vi "Callback - SpeechRecongized.vi"(4 "识别结果":refnum<vi>, 5 "事件数据":T1, 6 "控件引用":refnum<k24>, 7 "事件通用数据":cluster{"源":i32, "类型":u32, "时间":u32}) -> ()   [LabVIEW 2020]
doc: "该回调VI在网页浏览器ActiveX对象上运行Navigate2方法时运行。"
uses:
  System.Speech
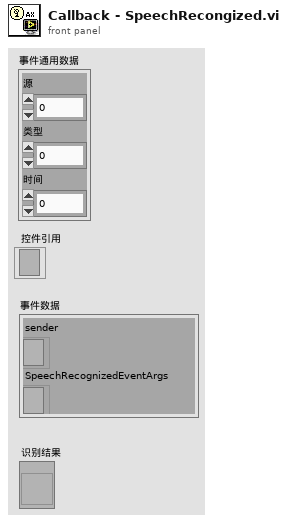
[diagram p1: front panel]
types:
  T1 = cluster{"sender":refnum<k24>, "SpeechRecognizedEventArgs":refnum<k24>}
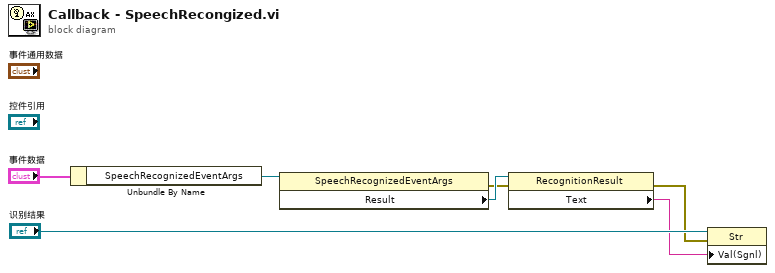
[diagram p0: block diagram]
diagram:
  n1 = Unbundle By Name("事件数据") -> ("SpeechRecognizedEventArgs"=w5:refnum<k24>)
  n2 = property class="SpeechRecognizedEventArgs"(reference=w5) -> (error out=w2:errorcluster, "Result"=w4:refnum<k24>)  [unwired: 1 in, 1 out]
  n3 = property class="RecognitionResult"(reference=w4, error in=w2) -> (error out=w1:errorcluster, "Text"=w3:string)  [unwired: 1 out]
  n4 = property class="Str"(reference="识别结果", error in=w1, "Val(Sgnl)"=w3) -> ()  [unwired: 2 out]
